vi "ReadArea.vi"() -> ()   [LabVIEW 2018]
uses:
  lib/Snap7.lvlib
panel:
  out "x-y":u32
  out "?":string
  out "ASCII Data":string
  out "Hex Data":string
  out "Running":bool
  out "Status":string="No Error"
  in  "Word Length":i32(ring)=2 items=["Bit"=1, "Byte"=2, "Word"=4, "DWord"=6, "Real"=8, "Counter"=28, "Timer"=29]
  in  "Area":i32(ring)=132 items=["Inputs (EB)"=129, "Output (AB)"=130, "Bit Memory (M)"=131, "Data (DB)"=132, "Counters (Z)"=28, "Timers (T)"=29]
  in  "Amount":i32=16
  in  "Start":i32
  in  "DB Number":i32=1
  out "Data":u8[](array[numeric])
  in  "?":bool
  in  "Slot":i32=2
  in  "Rack":i32
  in  "Address IP":string="192.168.1.12"
  # "Data Read"
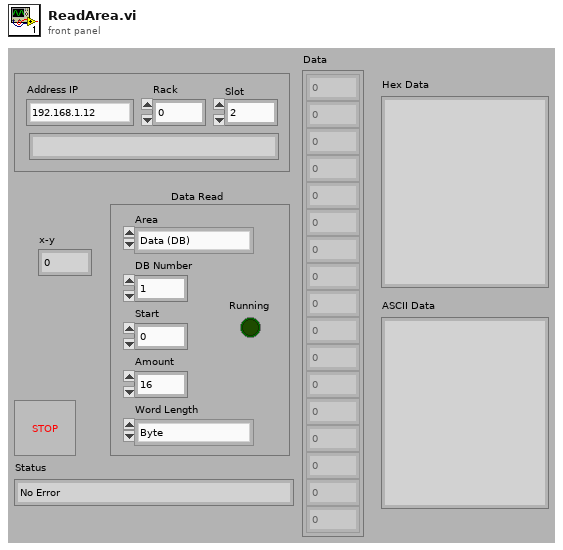
[diagram p1: front panel]
types:
  T1 = enum16{"big-endian, network order", "native, host order", "little-endian"}
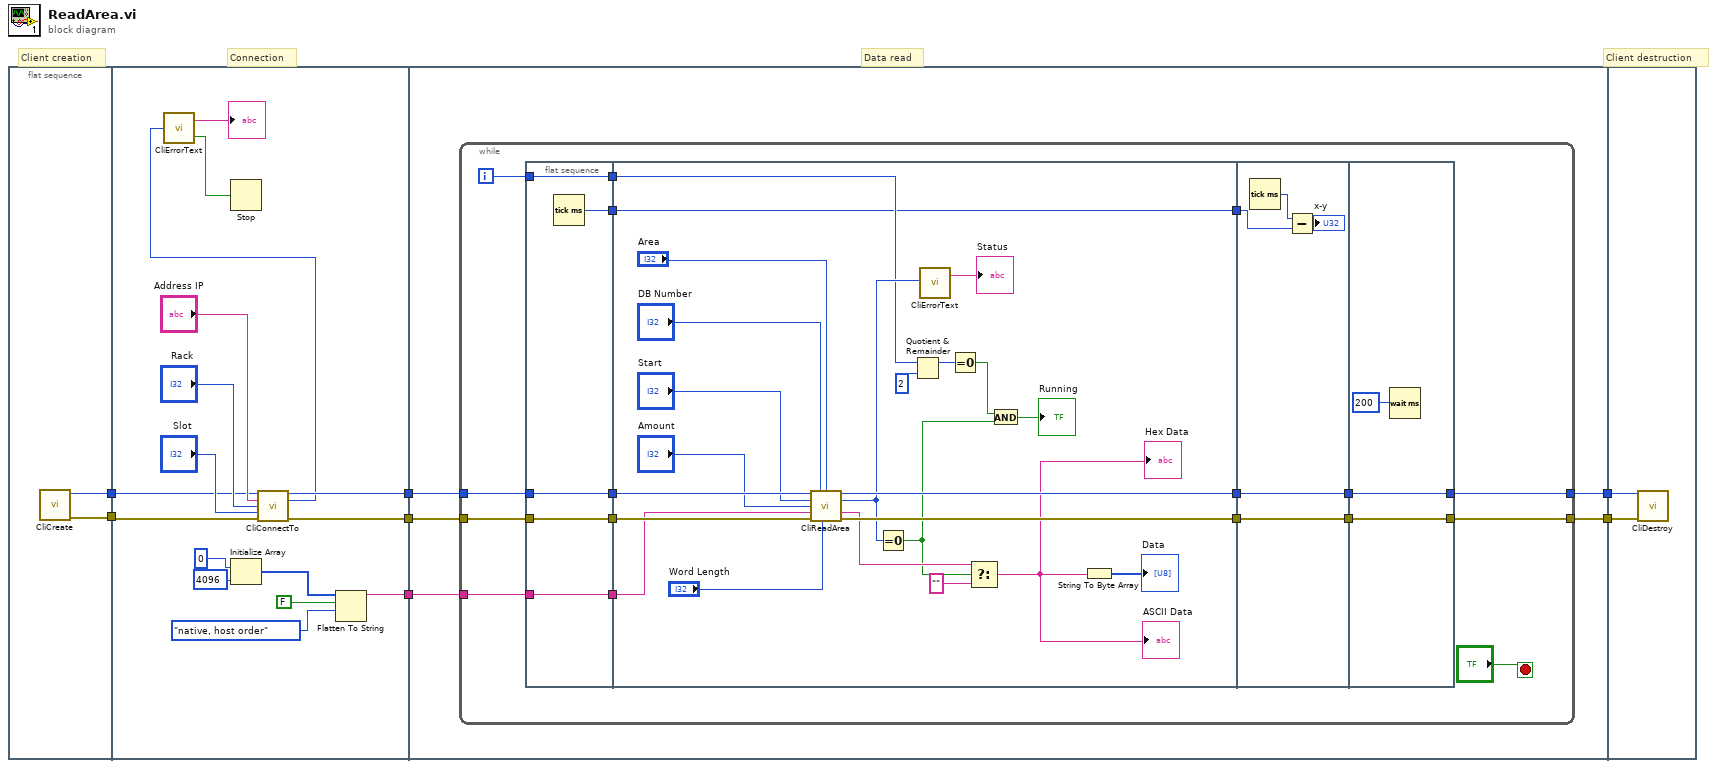
[diagram p0: block diagram]
diagram:
  # "Client destruction"
  # "Data read"
  # "Connection"
  # "Client creation"
  n1 = flat-sequence {
    tunnel: [w9] -> w4
    tunnel: [w8] -> w3
    tunnel: [w20] -> w7
    tunnel: [w13] -> w6
    tunnel: [w19] -> w5
    tunnel: w4 -> [w15]
    tunnel: w3 -> [w14]
    tunnel: w7 -> [w30]
    tunnel: w6 -> [w29]
    tunnel: w5 -> [w28]
    tunnel: [w27] -> w2
    tunnel: [w26] -> w1
    tunnel: w2 -> [w85]
    tunnel: w1 -> [w84]
    frame #0 {
      n2 = call "CliCreate.vi"() -> ("ref out"=w9:u64, "error out"=w8:errorcluster)  [unwired: 14 in]
    }
    frame #1 {
      n3 = Initialize Array(u8 0, 4096) -> (w23:u8[])
      n4 = call "CliConnectTo.vi"("ref in"=w15, "Address"="Address IP", "Rack"="Rack", "Slot"="Slot", "error in (no error)"=w14) -> ("ref out"=w13:u64, "Result"=w10:i32, "error out"=w20:errorcluster)  [unwired: 8 in]
      n5 = call "CliErrorText.vi"("ErrNo"=w10) -> ("Error"=w11:bool, "ErrMessage"=→"?":string)
      n6 = Stop(stop? (T)=w11) -> ()
      n7 = Flatten To String(anything=w23, prepend array or string size? (T)=FALSE, byte order (0:big-endian, network order)=T1."native, host order") -> (data string=w19:string)  [unwired: 1 in, 2 out]
    }
    frame #2 {
      n8 = while {
        tunnel: w30 -> [w46]
        tunnel: w29 -> [w45]
        tunnel: w28 -> [w44]
        tunnel: [w43] -> w27
        tunnel: [w42] -> w26
        i -> [w41]
        stop <- "?" stop-if-true
        n9 = flat-sequence {
          tunnel: w41 -> [w49]
          tunnel: w44 -> [w50]
          tunnel: w45 -> [w51]
          tunnel: w46 -> [w52]
          tunnel: [w52] -> w40
          tunnel: [w51] -> w39
          tunnel: [w50] -> w38
          tunnel: [w49] -> w37
          tunnel: [w48] -> w32
          tunnel: [w67] -> w36
          tunnel: [w66] -> w34
          tunnel: w40 -> [w75]
          tunnel: w39 -> [w74]
          tunnel: w38 -> [w73]
          tunnel: w37 -> [w64]
          tunnel: w32 -> [w53]
          tunnel: [w53] -> w31
          tunnel: w36 -> [w80]
          tunnel: [w80] -> w35
          tunnel: w34 -> [w79]
          tunnel: [w79] -> w33
          tunnel: w31 -> [w76]
          tunnel: [w82] -> w42
          tunnel: [w83] -> w43
          tunnel: w35 -> [w83]
          tunnel: w33 -> [w82]
          frame #0 {
            n10 = Tick Count (ms)() -> (millisecond timer value=w48:u32)
          }
          frame #1 {
            n11 = call "CliReadArea.vi"("ref in"=w74, "DB Number"="DB Number", "Area"="Area", "Start"="Start", "Amount"="Amount", "data in"=w73, "error in (no error)"=w75, "Word Length"="Word Length") -> ("ref out"=w67:u64, "Result"=w65:i32, "data out"=w58:string, "error out"=w66:errorcluster)  [unwired: 4 in]
            n12 = Equal To 0?(x=w65) -> (x = 0?=w57:bool)
            n13 = Quotient & Remainder(x=w64, y=2) -> (x-y*floor(x/y)=w62:i32)  [unwired: 1 out]
            n14 = call "CliErrorText.vi"("ErrNo"=w65) -> ("ErrMessage"=→"Status":string)  [unwired: 1 out]
            n15 = Equal To 0?(x=w62) -> (x = 0?=w61:bool)
            n16 = Select(t=w58, s=w57, f="") -> (s? t:f=w55:string)
            "ASCII Data" <- w55
            "Hex Data" <- w55
            n17 = And(x=w61, y=w57) -> (x .and. y?=→"Running":bool)
            n18 = String To Byte Array(string=w55) -> (unsigned byte array=→"Data":u8[])
          }
          frame #2 {
            n19 = Tick Count (ms)() -> (millisecond timer value=w77:u32)
            n20 = Subtract(x=w77, y=w76) -> (x-y=→"x-y":u32)
          }
          frame #3 {
            n21 = Wait (ms)(milliseconds to wait=u32 200 ("Loop Delay (ms)")) -> ()  [unwired: 1 out]
          }
        }
      }
    }
    frame #3 {
      n22 = call "CliDestroy.vi"("ref in"=w85, "error in (no error)"=w84) -> ()  [unwired: 13 in, 1 out]
    }
  }
